vi "array -- incert after.vi"(6 "index":i32, 8 "Array":dbl[](array[numeric]), 10 "number":dbl) -> (0 "array out":dbl[](array[numeric]), 1 "new index":i32)   [LabVIEW 2015]
uses:
  Q - not nan -- integer.vi
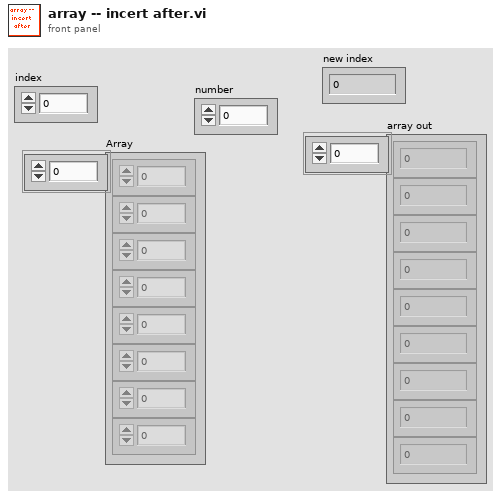
[diagram p1: front panel]
types:
  T1 = typedef "comparison control.ctl" = enum16{"not a number", "above", "in range", "below"}
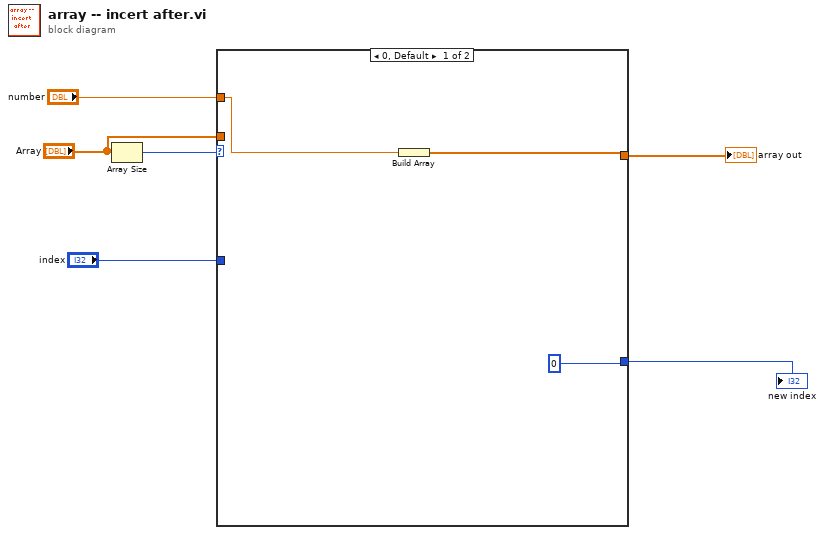
[diagram p0: block diagram]
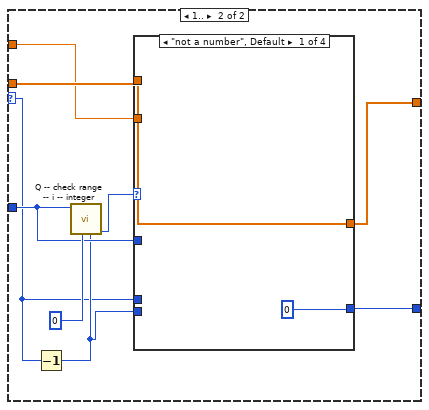
[diagram p2: hidden frame]
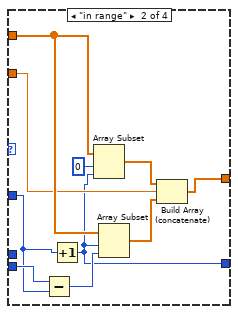
[diagram p3: hidden frame]
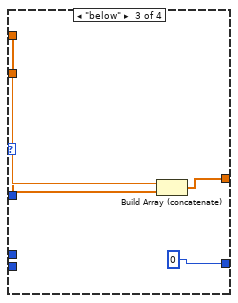
[diagram p4: hidden frame]
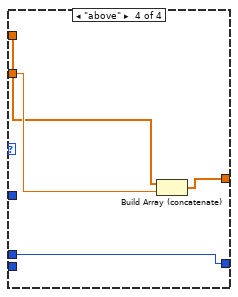
[diagram p5: hidden frame]
diagram:
  n1 = Array Size(array="Array") -> (size(s)=w6:i32)
  n2 = case shown="0, Default" w6 {
    selector: w6 -> [_ w10]
    tunnel: "number" -> [w9 w12]
    tunnel: [w8 w15] -> w4
    tunnel: "index" -> [_ w14]
    tunnel: "Array" -> [_ w18]
    tunnel: [0 w11] -> w1
    frame 0, Default {
      n3 = Build Array(w9) -> (w8:dbl[])
    }
    frame 1.. {
      n4 = Decrement(x=w10) -> (x-1=w13:i32)
      n5 = call "Q -- check range -- i -- integer.vi"("upper"=w13, "lower"=0, "number"=w14) -> ("selector"=w16:T1)  [unwired: 6 in, 2 out]
      n6 = case shown="\"not a number\", Default" w16 {
        tunnel: w18 -> [w20 w29 w32 w36]
        tunnel: [w20 w22 w34 w38] -> w15
        tunnel: w14 -> [_ w26 _ _]
        tunnel: w13 -> [_ w28 _ _]
        tunnel: w12 -> [_ w23 w33 w37]
        tunnel: [0 w21 0 w35] -> w11
        tunnel: w10 -> [_ _ _ w35]
        frame "not a number", Default {
        }
        frame "in range" {
          n7 = Subtract(x=w28, y=w26) -> (x-y=w27:i32)
          n8 = Increment(x=w26) -> (x+1=w21:i32)
          n9 = Array Subset(array=w29, index=0, length=w21) -> (w25:dbl[])
          n10 = Array Subset(array=w29, index=w21, length=w27) -> (w24:dbl[])
          n11 = Build Array (concatenate)(w25, w23, w24) -> (w22:dbl[])
        }
        frame "below" {
          n12 = Build Array (concatenate)(w33, w32) -> (w34:dbl[])
        }
        frame "above" {
          n13 = Build Array (concatenate)(w36, w37) -> (w38:dbl[])
        }
      }
    }
  }
  "array out" <- w4
  "new index" <- w1
